vi "Set Shop Floor System.vi"(8 "error in (no error)":errorcluster, 10 "Shop Floor System":refnum<class "Shop Floor System.lvclass">, 11 "App Properties in":refnum<class "App Properties.lvclass">) -> (0 "error out":errorcluster, 3 "App Properties out":refnum<class "App Properties.lvclass">)   [LabVIEW 2017]
uses:
  App Properties.lvclass
  C:/Program Files (x86)/National Instruments/LabVIEW 2017/vi.lib/TSS/ACRObat Test Framework/Classes/Base Objects/Base Class/Base Class/Class Properties/Class Properties.lvclass
  Shop Floor System/Class/Shop Floor System.lvclass
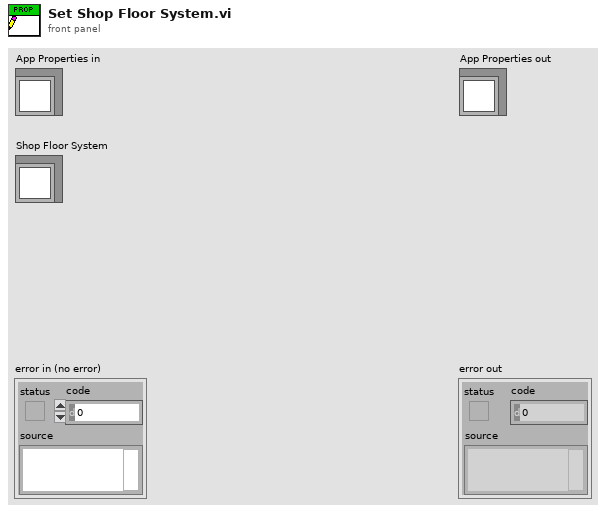
[diagram p1: front panel]
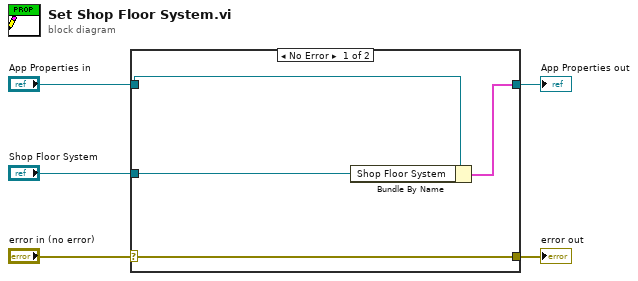
[diagram p0: block diagram]
diagram:
  n1 = case shown="No Error" "error in (no error)" {
    selector: "error in (no error)" -> [w9 w10]
    tunnel: [w9 w10] -> w4
    tunnel: [w7 w11] -> w2
    tunnel: "App Properties in" -> [w8 w11]
    tunnel: "Shop Floor System" -> [w6 _]
    frame No Error {
      n2 = Bundle By Name(cluster=w8, "Shop Floor System"=w6) -> (w7:cluster{})
    }
    frame Error {
    }
  }
  "error out" <- w4
  "App Properties out" <- w2
